vi "create_new_vi.vi"() -> (0 "error out":errorcluster, 3 "vi id":string)   [LabVIEW 2026]
doc: "Creates a new LabVIEW VI and shows the block diagram to the user. Use the returned vi id with other tools to modify the VI."
uses:
  G-AI Core.lvlib
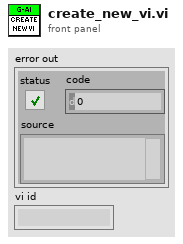
[diagram p1: front panel]
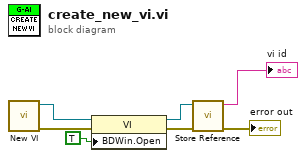
[diagram p0: block diagram]
diagram:
  n1 = call "New VI.vi"() -> ("error out"=w7:errorcluster, "VI Refnum"=w6:refnum<vi>)  [unwired: 10 in]
  n2 = property class="VI"(reference=w6, error in=w7, "BDWin.Open"=TRUE ("Block Diagram Window:Open")) -> (reference out=w3:refnum<vi>, error out=w4:errorcluster)
  n3 = call "Store Reference.vi"("error in"=w4, "Reference"=w3) -> ("error out"=→"error out":errorcluster, "id"=→"vi id":string)  [unwired: 8 in]
